vi "GPSMODBUSTCP解析.vi"(11 "Registers":u16[](array[numeric])) -> (3 "GPS解析":T1={"定位状态"=TRUE, "卫星数量"=0, "时间标识"=timestamp(0 s since 1904-01-01), "纬度"=0.0, "南北"="", "经度"=0.0, "东西"=""})   [LabVIEW 2016, in "环境动力监测库.lvlib" / "NMEA.lvlib"]
uses:
  NMEA.lvlib
  <vilib>/Utility/miscctls.llb/LVDateTimeRec.ctl
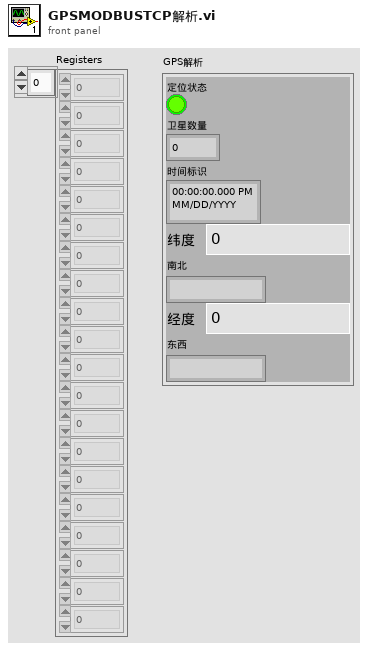
[diagram p1: front panel]
types:
  T1 = cluster{"定位状态":bool, "卫星数量":u16, "时间标识":timestamp, "纬度":dbl, "南北":string, "经度":dbl, "东西":string}
  T2 = typedef "LVDateTimeRec.ctl" = cluster{"fractional second":dbl, "second":i32, "minute":i32, "hour":i32, "day of month":i32, "month":i32, "year":i32, "day of week":i32, "day of year":i32, "DST":i32}
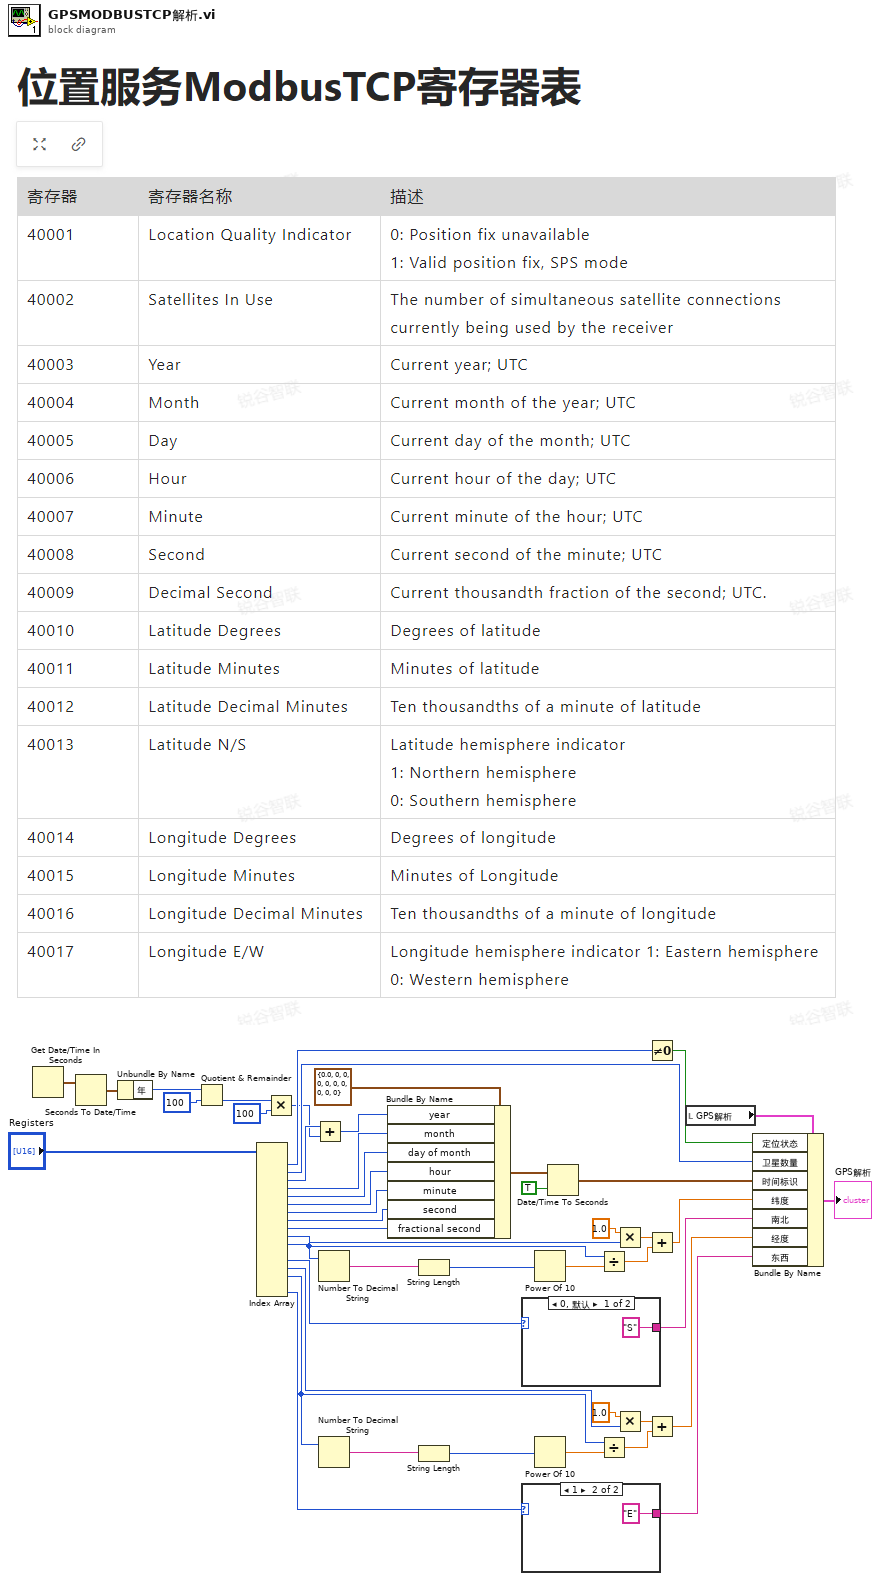
[diagram p0: block diagram]
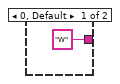
[diagram p2: hidden frame]
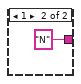
[diagram p3: hidden frame]
diagram:
  n1 = Get Date/Time In Seconds() -> (seconds since 1Jan1904=w29:timestamp)
  n2 = Seconds To Date/Time(time stamp (now)=w29) -> (date time rec=w28:T2)  [unwired: 1 in]
  n3 = Unbundle By Name(w28) -> ("年"=w27:i32)
  n4 = Quotient & Remainder(x=w27, y=100) -> (floor(x/y)=w25:i32)  [unwired: 1 out]
  n5 = Index Array(array="Registers") -> (element #1=w46:u16, element #2=w42:u16, element #3=w31:u16, element #4=w40:u16, element #5=w38:u16, element #6=w37:u16, element #7=w36:u16, element #8=w35:u16, element #9=w34:u16, element #10=w21:u16, element #11=w18:u16, element #13=w12:u16, element #14=w5:u16, element #15=w1:u16, element #17=w4:u16)  [unwired: 17 in, 2 out]
  n6 = Multiply(x=w25, y=100) -> (x*y=w23:i32)
  n7 = Add(x=w31, y=w23) -> (x+y=w30:i32)
  n8 = Number To Decimal String(number=w18) -> (decimal integer string=w19:string)  [unwired: 1 in]
  n9 = Number To Decimal String(number=w1) -> (decimal integer string=w8:string)  [unwired: 1 in]
  n10 = Bundle By Name(cluster=T2 {"fractional second"=0.0, "second"=0, "minute"=0, "hour"=0, "day of month"=0, "month"=0, "year"=0, "day of week"=0, "day of year"=0, "DST"=0} ("日期时间记录"), "year"=w30, "month"=w40, "day of month"=w38, "hour"=w37, "minute"=w36, "second"=w35, "fractional second"=w34) -> (w33:T2)
  n11 = String Length(string=w19) -> (length=w15:i32)
  n12 = String Length(string=w8) -> (length=w10:i32)
  n13 = case shown="0, 默认" w12 {
    tunnel: ["S" "N"] -> w13
    frame 0, Default {
    }
    frame 1 {
    }
  }
  n14 = case shown="1" w4 {
    tunnel: ["W" "E"] -> w2
    frame 0, Default {
    }
    frame 1 {
    }
  }
  n15 = Power Of 10(x=w15) -> (10^x=w14:dbl)
  n16 = Power Of 10(x=w10) -> (10^x=w11:dbl)
  n17 = Date/Time To Seconds(1:TRUE ("是UTC (F)"), 2:w33) -> (0:w32:timestamp)
  n18 = Divide(x=w18, y=w14) -> (x/y=w17:dbl)
  n19 = Divide(x=w1, y=w11) -> (x/y=w9:dbl)
  n20 = Multiply(x=1.0, y=w21) -> (x*y=w20:dbl)
  n21 = Multiply(x=1.0, y=w5) -> (x*y=w7:dbl)
  n22 = Not Equal To 0?(x=w46) -> (x != 0?=w44:bool)
  n23 = Add(x=w20, y=w17) -> (x+y=w16:dbl)
  n24 = Add(x=w7, y=w9) -> (x+y=w3:dbl)
  n25 = local read "GPS解析"() -> (w45:T1)
  n26 = Bundle By Name(cluster=w45, "定位状态"=w44, "卫星数量"=w42, "时间标识"=w32, "纬度"=w16, "南北"=w13, "经度"=w3, "东西"=w2) -> (→"GPS解析":T1)
